vi "SerializeMessage.vi"(7 "MsgSerializer":refnum<class "MsgSerializer.lvclass">, 9 "error in (no error)":errorcluster, 10 "Value":variant, 11 "TestManagerMsg in":refnum<class "TestManagerMsg.lvclass">) -> (1 "error out":errorcluster, 3 "Serialized Message":string)   [LabVIEW 2020, in "Caraya.lvlib" / "TestManagerMsg.lvclass"]
uses:
  TestManagerMsg.lvclass
  MsgSerializer/MsgSerializer.lvclass
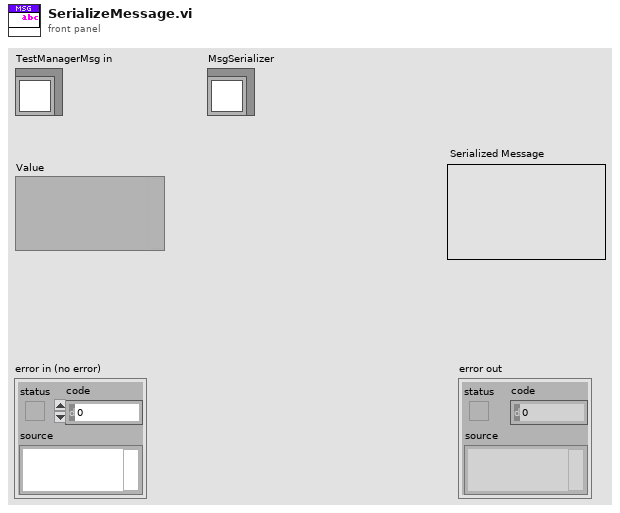
[diagram p1: front panel]
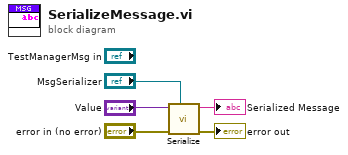
[diagram p0: block diagram]
diagram:
  n1 = call-dynamic "Serialize.vi"("MsgSerializer"="MsgSerializer", "error in (no error)"="error in (no error)", "Value"="Value") -> ("error out"=→"error out":errorcluster, "Serialized Message"=→"Serialized Message":string)  [unwired: 7 in]
